vi "iv from IV.vi"(8 "error in (no error)":errorcluster, 11 "IV_data in":refnum<class "IV_data.lvclass">) -> (0 "error out":errorcluster, 1 "y":dbl, 2 "x":dbl, 3 "IV_data out":refnum<class "IV_data.lvclass">)   [LabVIEW 2014, in "IV_data.lvclass"]
uses:
  IV_data.lvclass
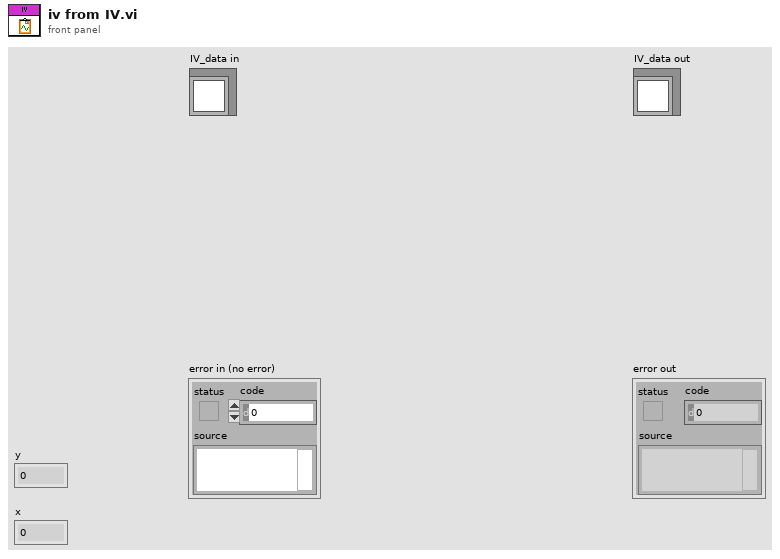
[diagram p1: front panel]
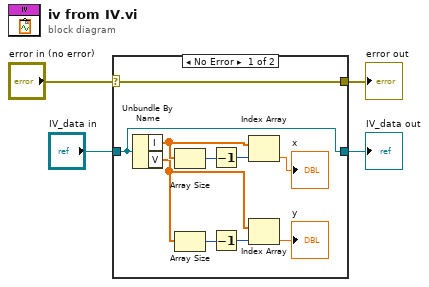
[diagram p0: block diagram]
diagram:
  n1 = case shown="No Error" "error in (no error)" {
    selector: "error in (no error)" -> [w5 w16]
    tunnel: "IV_data in" -> [w6 w15]
    tunnel: [w6 w15] -> w2
    tunnel: [w5 w16] -> w1
    frame No Error {
      n2 = Unbundle By Name(w6) -> ("I"=w10:dbl[], "V"=w9:dbl[])
      n3 = Array Size(array=w10) -> (size(s)=w13:i32)
      n4 = Array Size(array=w9) -> (size(s)=w11:i32)
      n5 = Decrement(x=w13) -> (x-1=w14:i32)
      n6 = Decrement(x=w11) -> (x-1=w12:i32)
      n7 = Index Array(array=w10, index=w14) -> (element=→"x":dbl)
      n8 = Index Array(array=w9, index=w12) -> (element=→"y":dbl)
    }
    frame Error {
    }
  }
  "error out" <- w1
  "IV_data out" <- w2
